vi "CMN_addstatusmessagevi.vi"(8 "error in (no error)":errorcluster, 11 "message  in":string) -> (0 "error out":errorcluster, 1 "TIMEOUT":bool, 2 "ERROR":bool, 3 "message out":string, 5 "modified message out":string)   [LabVIEW 2016]
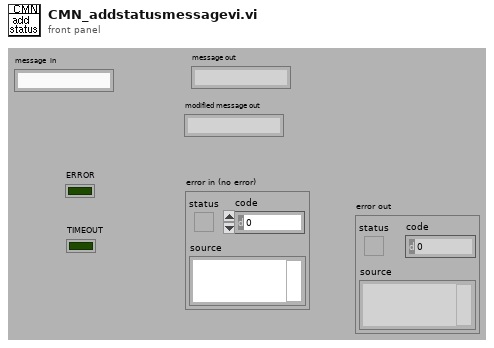
[diagram p1: front panel]
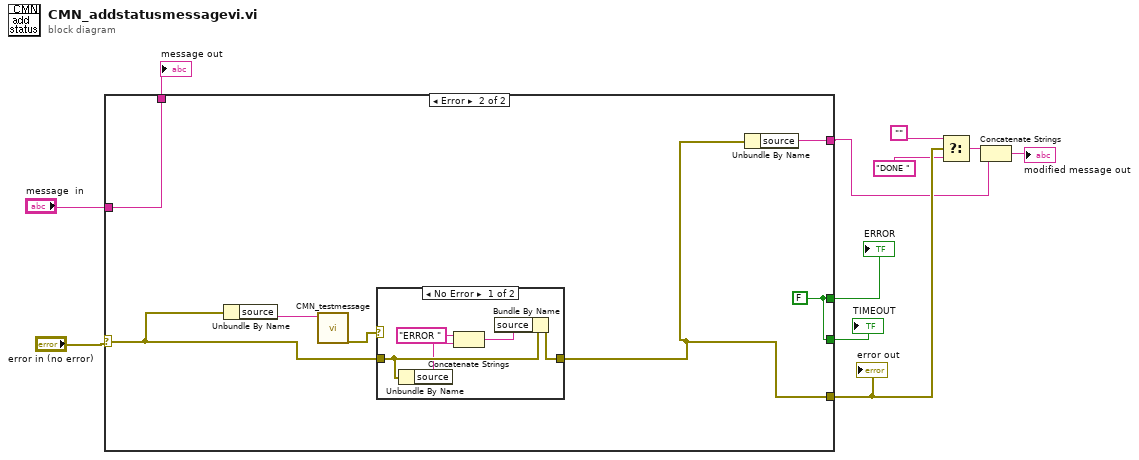
[diagram p0: block diagram]
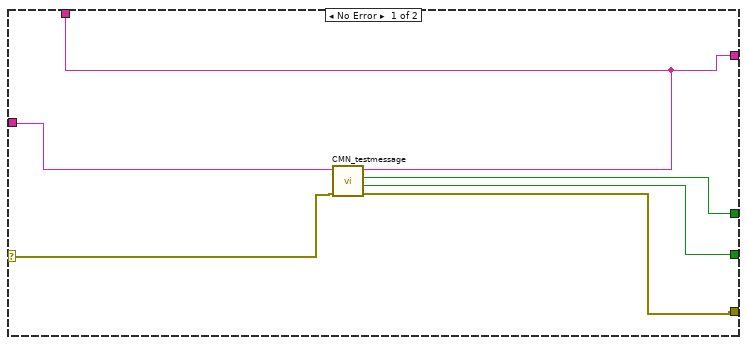
[diagram p2: hidden frame]
diagram:
  n1 = case shown="Error" "error in (no error)" {
    selector: "error in (no error)" -> [w12 w19]
    tunnel: [w13 w18] -> w8
    tunnel: [w14 w24] -> w10
    tunnel: [w15 w24] -> w9
    tunnel: [w16 w23] -> w5
    tunnel: "message  in" -> [w17 w22]
    tunnel: [w16 w22] -> w1
    frame No Error {
      n2 = call "CMN_testmessage.vi"("error in (no error)"=w12, "message  in"=w17) -> ("error out"=w13:errorcluster, "TIMEOUT"=w14:bool, "ERROR"=w15:bool, "message out"=w16:string)  [unwired: 6 out]
    }
    frame Error {
      w24 = FALSE
      n3 = Unbundle By Name(w19) -> ("source"=w21:string)
      n4 = call "CMN_testmessage.vi"("message  in"=w21) -> ("error out"=w20:errorcluster)  [unwired: 1 in, 9 out]
      n5 = case shown="No Error" w20 {
        tunnel: w19 -> [w28 w30]
        tunnel: [w29 w30] -> w18
        frame No Error {
          n6 = Unbundle By Name(w28) -> ("source"=w27:string)
          n7 = Concatenate Strings("ERROR " ("string"), w27) -> (w25:string)
          n8 = Bundle By Name(cluster=w28, "source"=w25) -> (w29:errorcluster)
        }
        frame Error {
        }
      }
      n9 = Unbundle By Name(w18) -> ("source"=w23:string)
    }
  }
  "error out" <- w8
  "ERROR" <- w9
  "TIMEOUT" <- w10
  "message out" <- w1
  n10 = Select(t="", s=w8, f="DONE ") -> (s? t:f=w7:string)
  n11 = Concatenate Strings(w7, w5) -> (→"modified message out":string)
